vi "MPExxx_init.vi"(2 "error in (no error)":errorcluster, 3 "ID Query (T: Query)":bool=TRUE, 4 "Reset Device (T: Reset)":bool=TRUE, 5 "VISA session":refnum<visa-resource-name>) -> (0 "error out":errorcluster {"code" format="%.0x"}, 1 "dup VISA session":refnum<visa-resource-name>)   [LabVIEW 2017]
doc: "This VI passes the addressing information in the instrument decriptor to the Instr Open VI and returns the instrument ID. You can optionally reset the instrument by setting the front panel reset control. You must run this VI before using any of the instrument driver VIs for this instrument."
uses:
  MPExxx Globals.gbl
panel:
  # "MAGNA-POWER"
  # "Electronics"
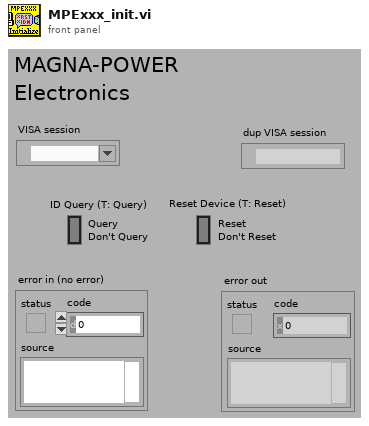
[diagram p1: front panel]
types:
  T1 = cluster{"Status":bool, "Code":i32, "Source (VI Name)":string}
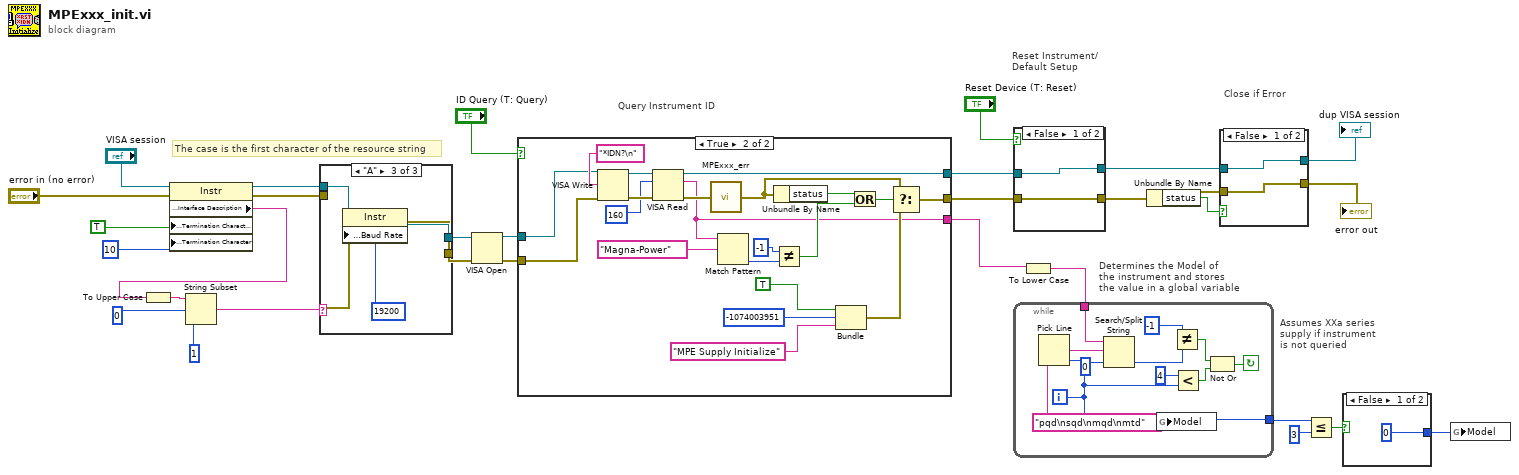
[diagram p0: block diagram]
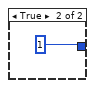
[diagram p2: hidden frame]
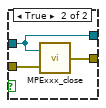
[diagram p3: hidden frame]
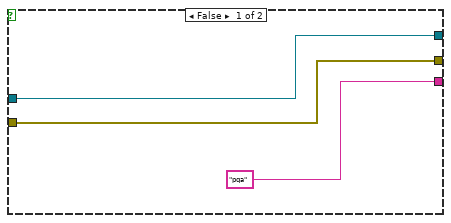
[diagram p4: hidden frame]
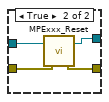
[diagram p5: hidden frame]
diagram:
  # "Assumes XXa series\nsupply if instrument\nis not queried"
  # "Determines the Model of\nthe instrument and stores\nthe value in a global variable"
  # "Close if Error"
  # "Reset Instrument/\nDefault Setup"
  # "Query Instrument ID"
  # "The case is the first character of the resource string"
  n1 = property class="Instr"(reference="VISA session", error in="error in (no error)", "Message Based Settings:Termination Character Enable"=TRUE, "Message Based Settings:Termination Character"=10) -> (reference out=w23:refnum<visa-resource-name>, error out=w22:errorcluster, "Interface Information:Interface Description"=w21:string)
  n2 = To Upper Case(1:w21) -> (0:w30:string)
  n3 = String Subset(string=w30, offset (0)=0, length (rest)=1) -> (substring=w29:string)
  n4 = case shown="\"A\"" w29 {
    tunnel: w23 -> [w31 w34 w39]
    tunnel: w22 -> [w32 w33 w38]
    tunnel: [w31 w34 w37] -> w16
    tunnel: [w32 w33 w36] -> w26
    frame "T", Default {
    }
    frame "G" {
    }
    frame "A" {
      n5 = property class="Instr"(reference=w39, error in=w38, "Serial Settings:Baud Rate"=19200) -> (reference out=w37:refnum<visa-resource-name>, error out=w36:errorcluster)
    }
  }
  n6 = VISA Open(error in (no error)=w26, VISA resource name=w16) -> (VISA resource name=w15:refnum<visa-resource-name>, error out=w14:errorcluster)  [unwired: 3 in]
  n7 = case shown="True" "ID Query (T: Query)" {
    tunnel: [w41 w55] -> w17
    tunnel: [w42 w60] -> w18
    tunnel: w15 -> [w42 w48]
    tunnel: w14 -> [w41 w47]
    tunnel: ["pqa" w43] -> w2
    frame False {
    }
    frame True {
      n8 = VISA Write(VISA resource name=w48, write buffer="*IDN?\n", error in (no error)=w47) -> (VISA resource name out=w58:refnum<visa-resource-name>, error out=w61:errorcluster)  [unwired: 1 out]
      n9 = VISA Read(VISA resource name=w58, byte count=u32 160, error in (no error)=w61) -> (VISA resource name out=w60:refnum<visa-resource-name>, read buffer=w43:string, error out=w46:errorcluster)  [unwired: 1 out]
      n10 = call "MPExxx_err.vi"("error in (no error)"=w46) -> ("error out"=w45:errorcluster)
      n11 = Match Pattern(string=w43, regular expression="Magna-Power") -> (offset past match=w53:i32)  [unwired: 1 in, 3 out]
      n12 = Unbundle By Name(w45) -> ("status"=w56:bool)
      n13 = Not Equal?(x=-1, y=w53) -> (x != y?=w49:bool)
      n14 = Bundle("Status"=TRUE, "Code"=-1074003951, "Source (VI Name)"="MPE Supply Initialize") -> (w50:T1)  [unwired: 1 in]
      n15 = Or(x=w56, y=w49) -> (x .or. y?=w57:bool)
      n16 = Select(t=w45, s=w57, f=w50) -> (s? t:f=w55:T1)
    }
  }
  n17 = case shown="False" "Reset Device (T: Reset)" {
    tunnel: w17 -> [w64 w68]
    tunnel: [w64 w66] -> w10
    tunnel: w18 -> [w65 w69]
    tunnel: [w65 w67] -> w9
    frame False {
    }
    frame True {
      n18 = call "MPExxx_Reset.vi"("error in (no error)"=w68, "VISA session"=w69) -> ("error out"=w66:errorcluster, "dup VISA session"=w67:refnum<visa-resource-name>)
    }
  }
  n19 = To Lower Case(string=w2) -> (all lower case string=w1:string)
  n20 = while {
    tunnel: [w73] -> w4
    tunnel: w1 -> [w77]
    i -> [w73]
    stop <- w70 continue-if-true
    n21 = Pick Line(multi-line string="pqd\nsqd\nmqd\nmtd", line index=w73) -> (output string=w79:string)  [unwired: 1 in]
    n22 = Search/Split String(string=w77, search string/char (-)=w79, offset (0)=0) -> (offset of match=w75:i32)  [unwired: 2 out]
    n23 = global write "MPExxx Globals.gbl" "Model"(w73) -> ()
    n24 = Not Equal?(x=-1, y=w75) -> (x != y?=w71:bool)
    n25 = Less?(x=4, y=w73) -> (x < y?=w72:bool)
    n26 = Not Or(1:w72, 2:w71) -> (0:w70:bool)
  }
  n27 = Unbundle By Name(w10) -> ("status"=w11:bool)
  n28 = case shown="False" w11 {
    tunnel: w9 -> [w82 w83]
    tunnel: w10 -> [w81 w85]
    tunnel: [w82 w83] -> w8
    tunnel: [w81 w84] -> w7
    frame False {
    }
    frame True {
      n29 = call "MPExxx_close.vi"("error in (no error)"=w85, "VISA session"=w83) -> ("error out"=w84:errorcluster)
    }
  }
  "dup VISA session" <- w8
  "error out" <- w7
  n30 = Less Or Equal?(x=w4, y=3) -> (x <= y?=w5:bool)
  n31 = case shown="False" w5 {
    tunnel: [0 1] -> w6
    frame False {
    }
    frame True {
    }
  }
  n32 = global write "MPExxx Globals.gbl" "Model"(w6) -> ()
